vi "Write Measurement2D.lvclass.vi"(8 "error in (no error)":errorcluster, 10 "Measurement2D.lvclass":refnum<class "Measurement2D.lvclass">, 11 "Experiment2D in":refnum<class "Experiment2D.lvclass">) -> (0 "error out":errorcluster, 3 "Experiment2D out":refnum<class "Experiment2D.lvclass">)   [LabVIEW 2014, in "Experiment2D.lvclass"]
uses:
  Experiment2D.lvclass
  Measurement/Measurement2D/Measurement2D.lvclass
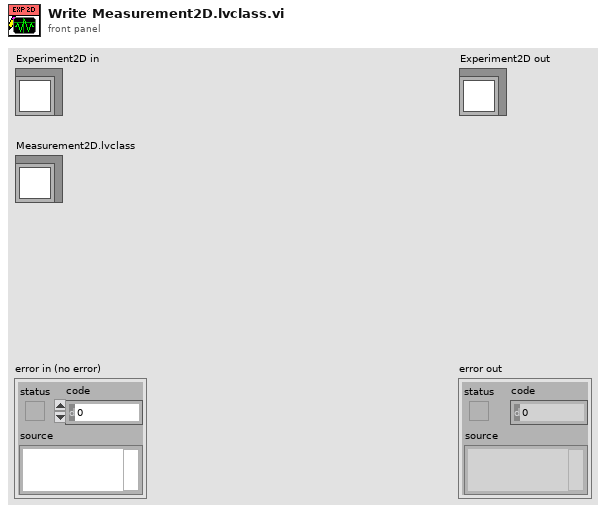
[diagram p1: front panel]
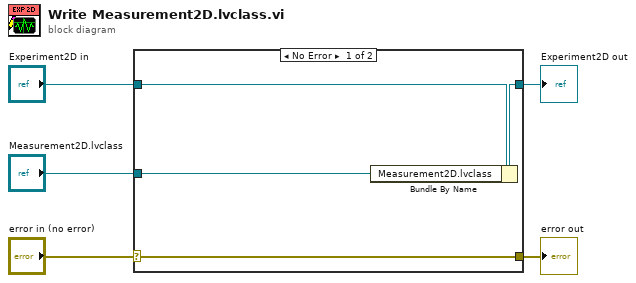
[diagram p0: block diagram]
diagram:
  n1 = case shown="No Error" "error in (no error)" {
    selector: "error in (no error)" -> [w9 w10]
    tunnel: [w9 w10] -> w4
    tunnel: [w7 w11] -> w2
    tunnel: "Experiment2D in" -> [w8 w11]
    tunnel: "Measurement2D.lvclass" -> [w6 _]
    frame No Error {
      n2 = Bundle By Name(cluster=w8, "Measurement2D.lvclass"=w6) -> (w7:refnum<class "Experiment2D.lvclass">)
    }
    frame Error {
    }
  }
  "error out" <- w4
  "Experiment2D out" <- w2
